vi "GLOBAL -MAIN.vi"() -> ()   [LabVIEW 2021]
panel:
  out "EXIT":bool
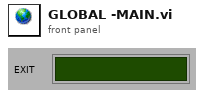
[diagram p1: front panel]
diagram:
